vi "Create Coverage Report.vi"(7 "Time Stamp (Now)":timestamp, 9 "Project Inspector":refnum<class "Project Inspector Base.lvclass">, 10 "Code Inspector":refnum<class "Code Inspector Base.lvclass">, 11 "CodeCoverage in":refnum<class "Code Coverage.lvclass">) -> (2 "Coverage":refnum<class "Coverage.lvclass">, 3 "CodeCoverage out":refnum<class "Code Coverage.lvclass">)   [LabVIEW 2017, in "Cobertura.lvlib"]
uses:
  Cobertura.lvlib
  Code Coverage/Code Coverage.lvclass
  Coverage/Coverage.lvclass
  Code Inspector Base/Code Inspector Base.lvclass
  Project Inspector Base/Project Inspector Base.lvclass
  Package/Package.lvclass
  Package/Package.lvclass/Package.ctl
  Package/Read Name.vi
  Class/Class.lvclass
  Method/Method.lvclass
  Line/Line.lvclass
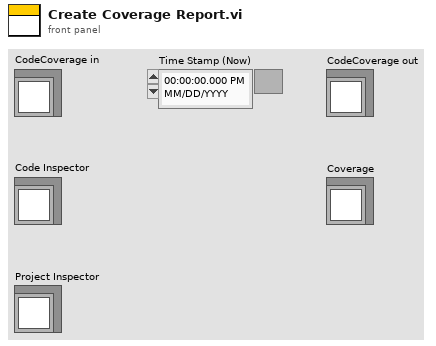
[diagram p1: front panel]
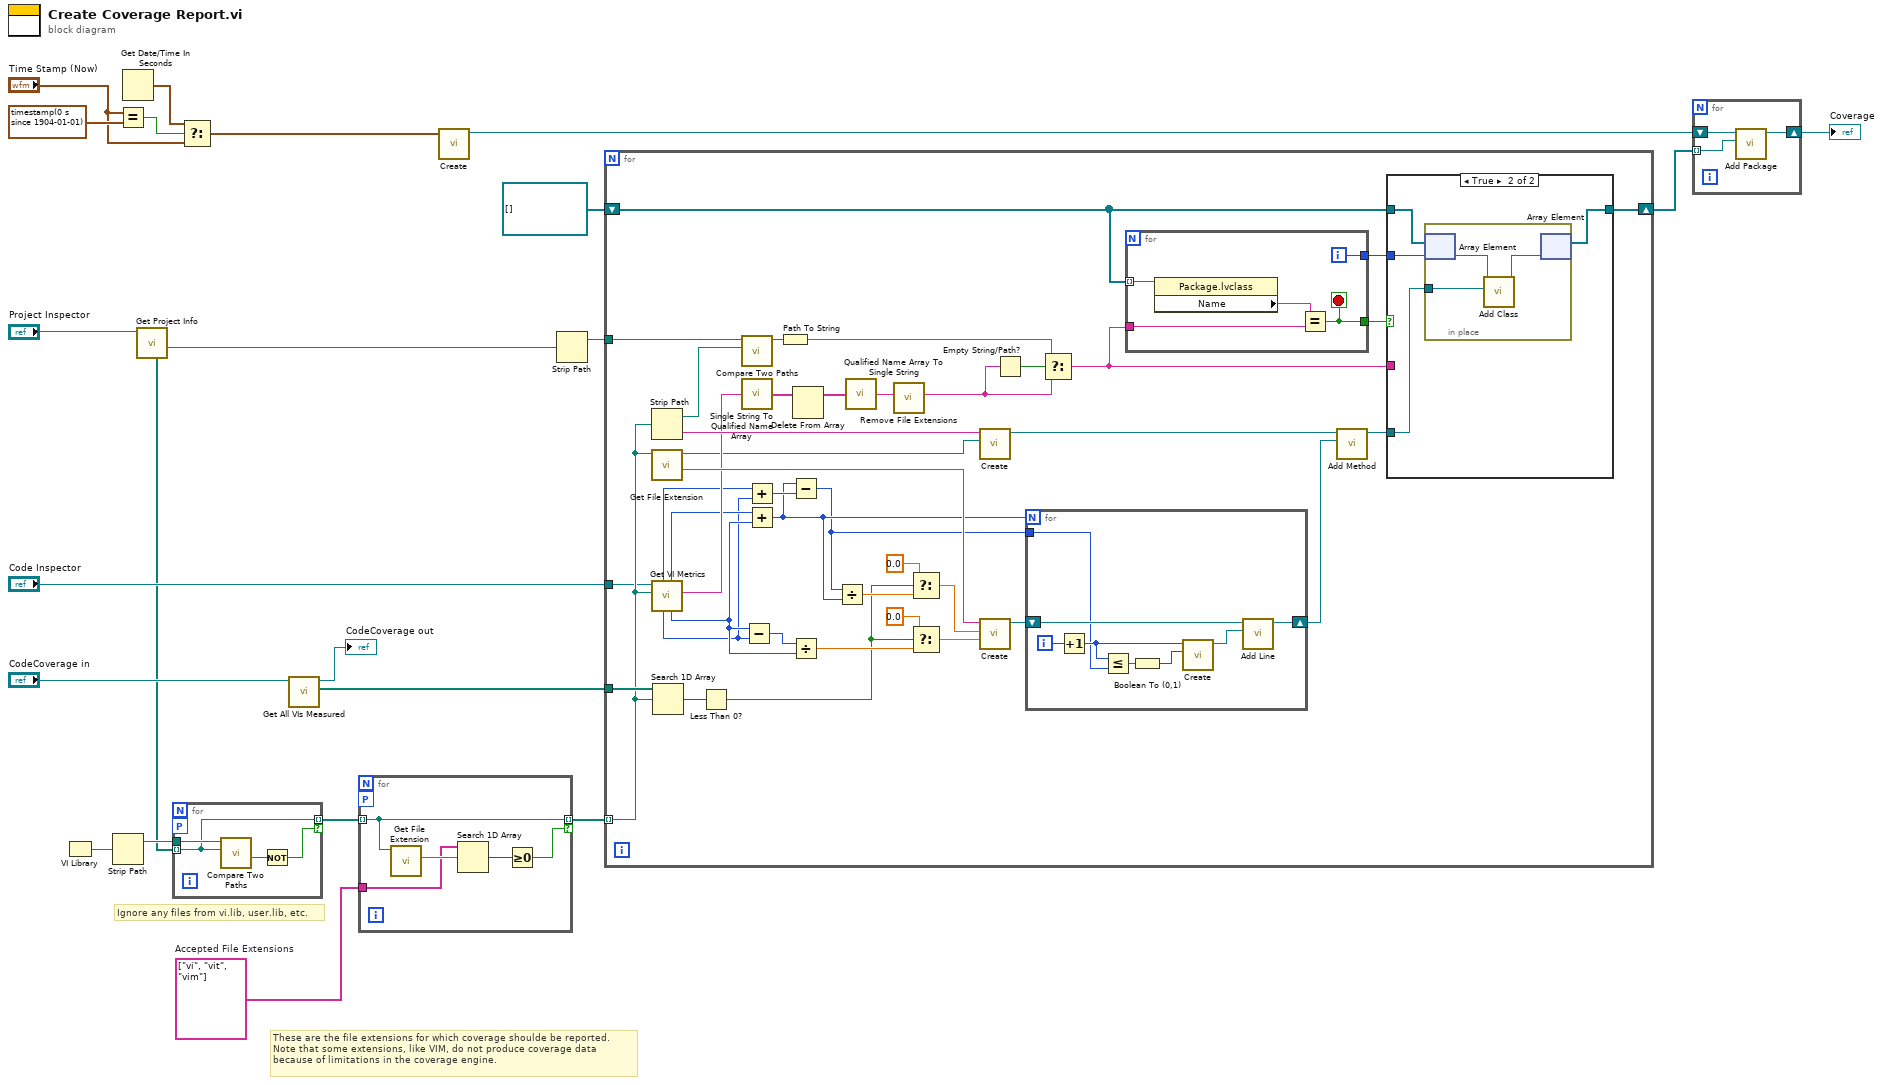
[diagram p0: block diagram]
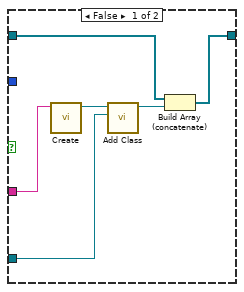
[diagram p2: hidden frame]
diagram:
  w2 = string[] ["vi", "vit", "vim"]  # Accepted File Extensions
  # "These are the file extensions for which coverage shoulde be reported.\nNote that some extensions, like VIM, do not produce coverage data\nbecause of limitations in the coverage engine."
  # "Ignore any files from vi.lib, user.lib, etc."
  n1 = VI Library() -> (path=w18:path)
  n2 = Strip Path(path=w18) -> (stripped path=w17:path)  [unwired: 1 out]
  n3 = Equal?(x="Time Stamp (Now)", y=timestamp(0 s since 1904-01-01) ("Time Stamp (Now)")) -> (x = y?=w8:bool)
  n4 = Get Date/Time In Seconds() -> (seconds since 1Jan1904=w7:timestamp)
  n5 = call-dynamic "Get Project Info.vi"("Project Inspector Base in"="Project Inspector") -> ("Path"=w11:path, "Item Paths"=w10:path[])  [unwired: 6 in, 3 out]
  n6 = for {
    tunnel: w10 -> [w23] mode=indexing
    tunnel: [w23] -> w3 mode=indexing if=w25
    tunnel: w17 -> [w24]
    workers-P: _ -> [_]
    n7 = call <vilib>:"Compare Two Paths.vi"("Path 2"=w23, "Path 1"=w24) -> ("Path 2 Relative to Path 1?"=w26:bool)  [unwired: 6 in, 3 out]
    n8 = Not(x=w26) -> (.not. x?=w25:bool)
  }
  n9 = Select(t=w7, s=w8, f="Time Stamp (Now)") -> (s? t:f=w5:timestamp)
  n10 = call-dynamic "Get All VIs Measured.vi"("CodeCoverage in"="CodeCoverage in") -> ("All VIs Measured"=w15:path[], "CodeCoverage out"=→"CodeCoverage out":refnum<class "Code Coverage.lvclass">)  [unwired: 8 in, 1 out]
  n11 = for {
    tunnel: w3 -> [w30] mode=indexing
    tunnel: [w30] -> w4 mode=indexing if=w31
    workers-P: _ -> [_]
    tunnel: w2 -> [w28]
    n12 = call <vilib>:"Get File Extension.vi"("file"=w30) -> ("lowercase file extension"=w29:string)  [unwired: 6 in, 4 out]
    n13 = Search 1D Array(1D array=w28, element=w29) -> (index of element=w27:i32)  [unwired: 1 in]
    n14 = Greater Or Equal To 0?(x=w27) -> (x >= 0?=w31:bool)
  }
  n15 = call "Create.vi"("Timestamp"=w5) -> ("Coverage"=w21:refnum<class "Coverage.lvclass">)  [unwired: 9 in, 1 out]
  n16 = Strip Path(path=w11) -> (stripped path=w14:path)  [unwired: 1 out]
  n17 = for {
    tunnel: "Code Inspector" -> [w42]
    shift-right: [w65] -> w20
    shift-left: refnum<class "Package.lvclass">[] [] -> [w68]
    tunnel: w4 -> [w43] mode=indexing
    tunnel: w15 -> [w57]
    tunnel: w14 -> [w44]
    n18 = Strip Path(path=w43) -> (stripped path=w46:path, name=w61:string)
    n19 = call <vilib>:"Get File Extension.vi"("file"=w43) -> ("filename without extension"=w62:string, "dup file"=w40:path)  [unwired: 6 in, 3 out]
    n20 = call-dynamic "Get VI Metrics.vi"("VI Path"=w43, "Code Inspector in"=w42) -> ("VI Name"=w41:string, "Total Diagram Count"=w37:i32, "Total Node Count"=w38:i32, "Uncovered Diagram Count"=w36:i32, "Uncovered Node Count"=w35:i32)  [unwired: 3 in, 2 out]
    n21 = Search 1D Array(1D array=w57, element=w43) -> (index of element=w56:i32)  [unwired: 1 in]
    n22 = Less Than 0?(x=w56) -> (x < 0?=w51:bool)
    n23 = call <vilib>:"Compare Two Paths.vi"("Path 2"=w46, "Path 1"=w44) -> ("Relative Path from 1 to 2"=w45:path)  [unwired: 6 in, 3 out]
    n24 = call <vilib>:"Single String To Qualified Name Array.vi"("Fully Qualified String"=w41) -> ("Fully Qualified Array"=w72:string[])
    n25 = Subtract(x=w37, y=w36) -> (x-y=w58:i32)
    n26 = Add(x=w35, y=w36) -> (x+y=w34:i32)
    n27 = Add(x=w38, y=w37) -> (x+y=w33:i32)
    n28 = Path To String(path=w45) -> (string=w39:string)
    n29 = Subtract(x=w33, y=w34) -> (x-y=w32:i32)
    n30 = Divide(x=w58, y=w37) -> (x/y=w53:dbl)
    n31 = Delete From Array(array=w72) -> (array with subset deleted=w71:string[])  [unwired: 2 in, 1 out]
    n32 = Divide(x=w32, y=w33) -> (x/y=w55:dbl)
    n33 = call <vilib>:"Qualified Name Array To Single String.vi"("Fully Qualified Array"=w71) -> ("Fully Qualified String"=w48:string)
    n34 = call "Remove File Extensions.vi"("String"=w48) -> ("String out"=w47:string)  [unwired: 10 in]
    n35 = Select(t=0.0, s=w51, f=w55) -> (s? t:f=w54:dbl)
    n36 = Select(t=0.0, s=w51, f=w53) -> (s? t:f=w52:dbl)
    n37 = call "Create.vi"("Filename"=w40, "Name"=w61) -> ("Class"=w64:refnum<class "Class.lvclass">)  [unwired: 8 in, 1 out]
    n38 = call "Create.vi"("Branch Rate"=w52, "Line Rate"=w54, "Name"=w62) -> ("Method"=w60:refnum<class "Method.lvclass">)  [unwired: 7 in, 1 out]
    n39 = Empty String/Path?(string/path=w47) -> (empty?=w70:bool)
    n40 = for {
      N: w33 -> [_]
      shift-right: [w75] -> w59
      shift-left: w60 -> [w74]
      tunnel: w32 -> [w73]
      i -> [w80]
      n41 = Increment(x=w80) -> (x+1=w79:i32)
      n42 = Less Or Equal?(x=w79, y=w73) -> (x <= y?=w78:bool)
      n43 = Boolean To (0,1)(Boolean=w78) -> (0, 1=w77:i16)
      n44 = call "Create.vi"("Hits"=w77, "Number"=w79) -> ("Line"=w76:refnum<class "Line.lvclass">)  [unwired: 8 in, 1 out]
      n45 = call "Add Line.vi"("Line"=w76, "Method in"=w74) -> ("Method out"=w75:refnum<class "Method.lvclass">)  [unwired: 8 in, 1 out]
    }
    n46 = Select(t=w39, s=w70, f=w47) -> (s? t:f=w66:string)
    n47 = for {
      tunnel: w68 -> [w98] mode=indexing
      tunnel: w66 -> [w96]
      tunnel: [w95] -> w69
      tunnel: [w94] -> w67
      i -> [w94]
      stop <- w95 stop-if-true
      n48 = property class="Package.lvclass"(reference=w98) -> ("Name"=w97:string)  [unwired: 1 in, 2 out]
      n49 = Equal?(x=w97, y=w96) -> (x = y?=w95:bool)
    }
    n50 = call "Add Method.vi"("Method"=w59, "Class in"=w64) -> ("Class out"=w63:refnum<class "Class.lvclass">)  [unwired: 8 in, 1 out]
    n51 = case shown="True" w69 {
      tunnel: w68 -> [w86 w90]
      tunnel: [w85 w89] -> w65
      tunnel: w63 -> [w82 w88]
      tunnel: w67 -> [_ w87]
      tunnel: w66 -> [w81 _]
      frame False {
        n52 = call "Create.vi"("Name"=w81) -> ("Package"=w84:refnum<class "Package.lvclass">)  [unwired: 9 in, 1 out]
        n53 = call "Add Class.vi"("Class"=w82, "Package in"=w84) -> ("Package out"=w83:refnum<class "Package.lvclass">)  [unwired: 8 in, 1 out]
        n54 = Build Array (concatenate)(w86, w83) -> (w85:refnum<class "Package.lvclass">[])
      }
      frame True {
        n55 = in-place {
          in-place-border: w88 -> [w91]
          n56 = in-place-array #1(w90, w87) -> (w93:refnum<class "Package.lvclass">)
          n57 = call "Add Class.vi"("Class"=w91, "Package in"=w93) -> ("Package out"=w92:refnum<class "Package.lvclass">)  [unwired: 8 in, 1 out]
          n58 = in-place-array #1(w92) -> (w89:refnum<class "Package.lvclass">[])  [unwired: 1 out]
        }
      }
    }
  }
  n59 = for {
    tunnel: w20 -> [w101] mode=indexing
    shift-right: [w100] -> w19
    shift-left: w21 -> [w99]
    n60 = call "Add Package.vi"("Package"=w101, "Coverage in"=w99) -> ("Coverage out"=w100:refnum<class "Coverage.lvclass">)  [unwired: 8 in, 1 out]
  }
  "Coverage" <- w19
